vi "Load and Execute Tests Process__core.vi"(0 "TestTag Argument":string, 1 "Operation":enum16{"Load", "Run Test", "Run All Tests"}(ring), 5 "TestStatusEvents":T1, 7 "AbortEvent":refnum<user-event>, 9 "TextStream":refnum<queue>, 11 "Test Hierarchy Tree ref":refnum<vi>, 12 "API_TextTestRunner":refnum<class>, 13 "Test Project":path, 14 "error in":errorcluster) -> (4 "Tree Methods":i32, 15 "error out":errorcluster)   [LabVIEW 2013, in "GraphicalTestRunner.lvlib"]
uses:
  GraphicalTestRunner.lvlib
  Classes/TestResult/resultStatusChanged--Cluster.ctl
  Classes/TestResult/resultStatus--enum.ctl
  Classes/TestSuite/suiteStatusChanged--Cluster.ctl
  Classes/TestSuite/suiteStatus--enum.ctl
  Classes/TestSuite/TestSuite.lvclass
  Classes/TextTestRunner/TextTestRunner.lvclass
  Classes/TestLoader/TestLoader.lvclass
  Classes/TestRunner/PublicEvents--Cluster.ctl
  Classes/TestResult/testStarted--Cluster.ctl
  <userlib>/_OpenG.lib/file/file.llb/Strip Path - Arrays__ogtk.vi
  <userlib>/_OpenG.lib/array/array.llb/Filter 1D Array (String)__ogtk.vi
  <userlib>/_OpenG.lib/array/array.llb/Delete Elements from 1D Array (Path)__ogtk.vi
  <userlib>/_OpenG.lib/array/array.llb/Conditional Auto-Indexing Tunnel (Path)__ogtk.vi
  Libraries/VITesterUtilities.lvlib
  Classes/TestResult/TestResult.lvclass
  Classes/TestRunner/TestRunner.lvclass
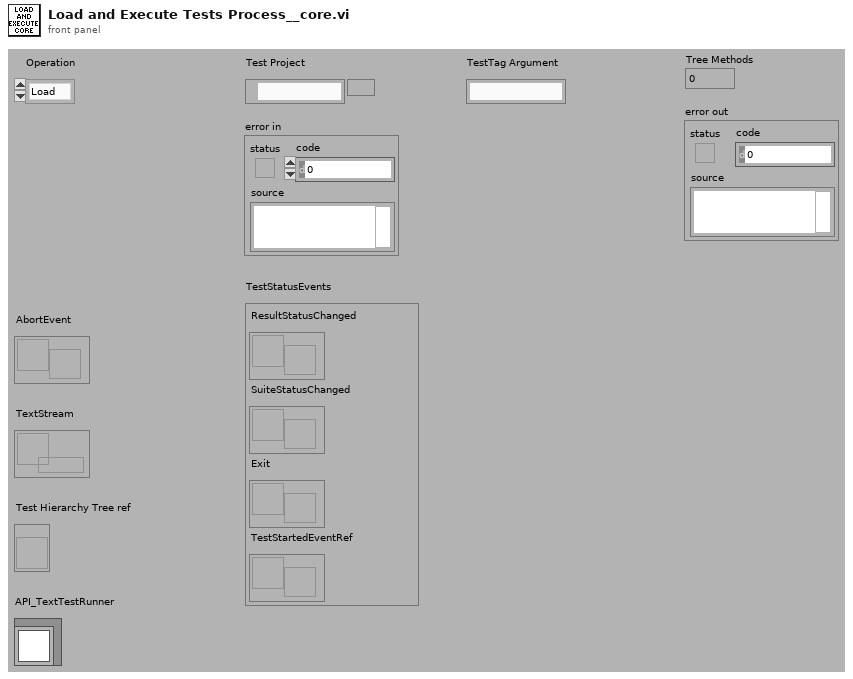
[diagram p1: front panel]
types:
  T1 = cluster{"ResultStatusChanged":refnum<user-event>, "SuiteStatusChanged":refnum<user-event>, "Exit":refnum<user-event>, "TestStartedEventRef":refnum<user-event>}
  T2 = cluster{"Current VI's Refnum":refnum<vi>, "menubar":refnum<k9>, "TextStream":refnum<queue>, "TestMethod":string, "Open Path":path, "Test Project":path, "TestProjectClasses":path[], "TestApplicationContext":refnum<vi>, "Test Class":path, "ResultChangedRef":refnum<user-event>, "SuiteChangedRef":refnum<user-event>, "TestTag":string, "AbortEventRef":refnum<user-event>, "ExitEventReference":refnum<user-event>, "AllTests.TestSuite":refnum<class "TestSuite.lvclass">, "error":errorcluster, "TextTestRunner":refnum<class "TextTestRunner.lvclass">, "TestStartedEventRef":refnum<user-event>}
  T3 = enum32{"Invalid", "Standard", "Closed", "Hidden", "Minimized", "Maximized"}
  T4 = typedef "TestRunner.lvclass/PublicEvents--Cluster.ctl" = cluster{"abortEventRef":refnum<user-event>, "resultStatusChangedEventRef":refnum<user-event>, "testStartedEventRef":refnum<user-event>}
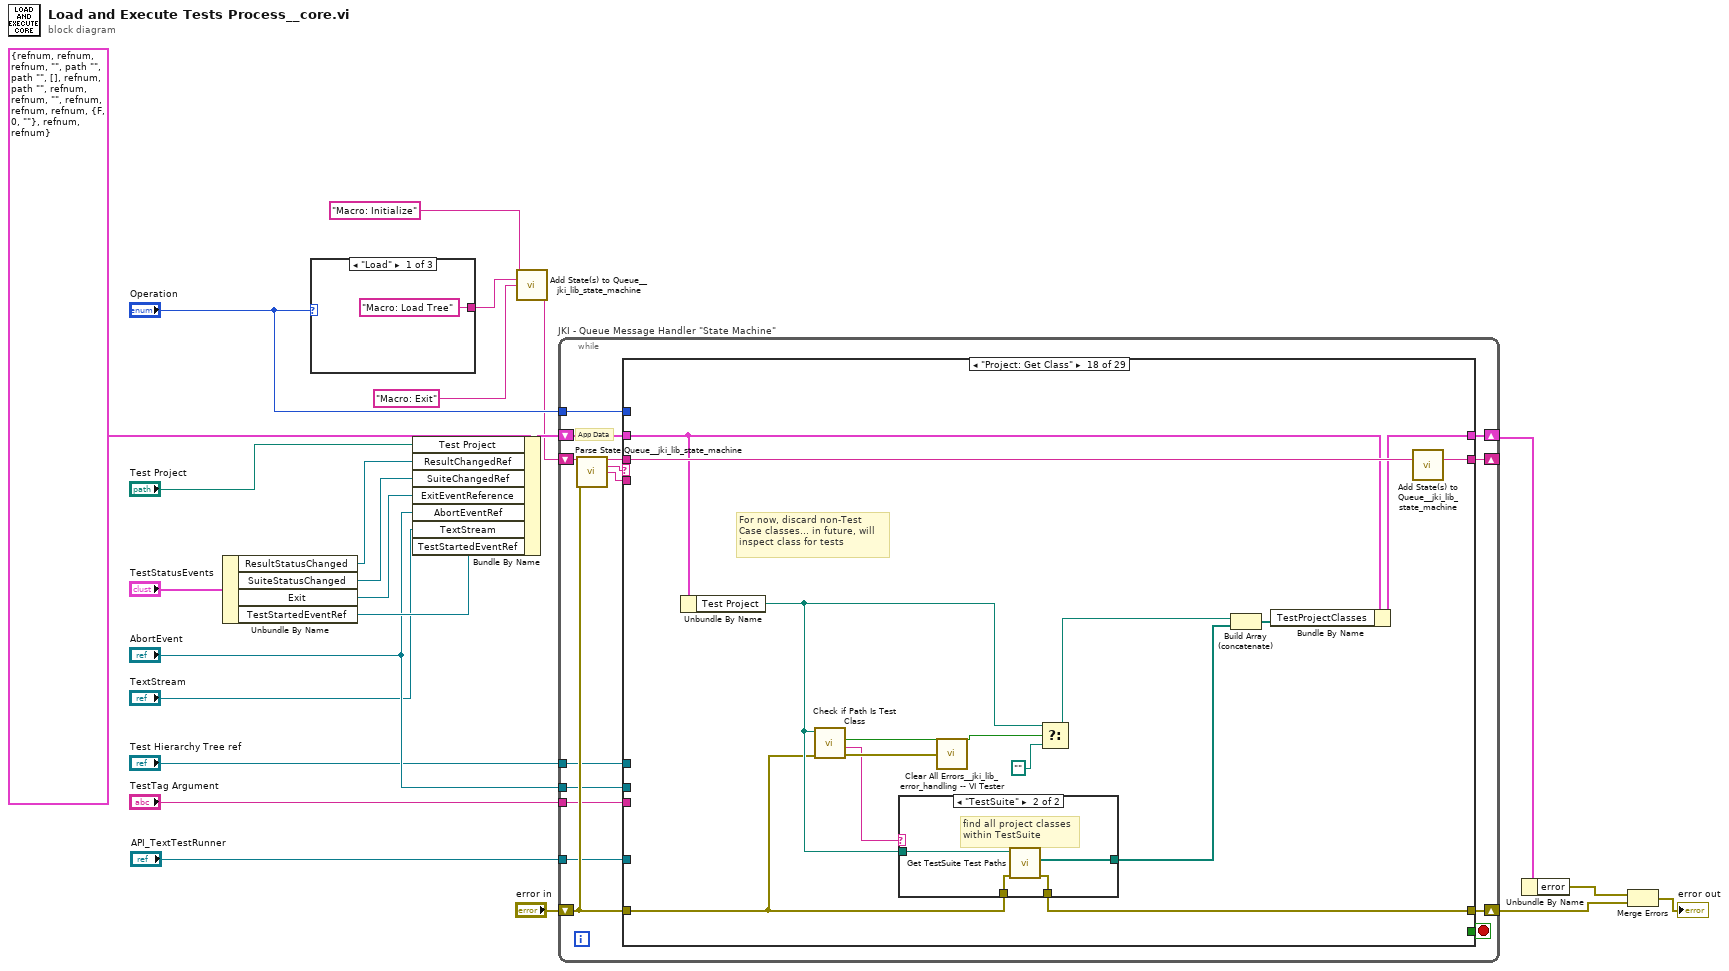
[diagram p0: block diagram]
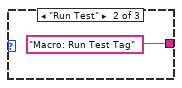
[diagram p2: hidden frame]
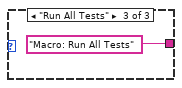
[diagram p3: hidden frame]
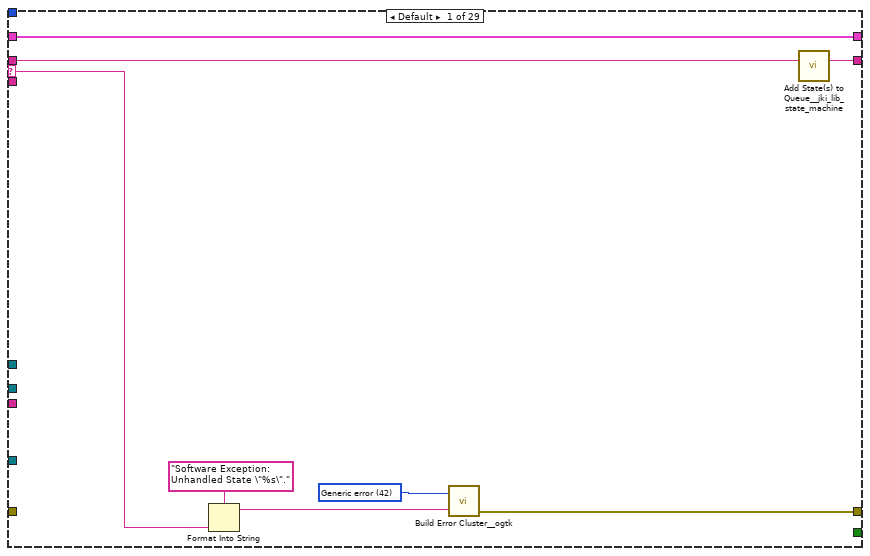
[diagram p4: hidden frame]
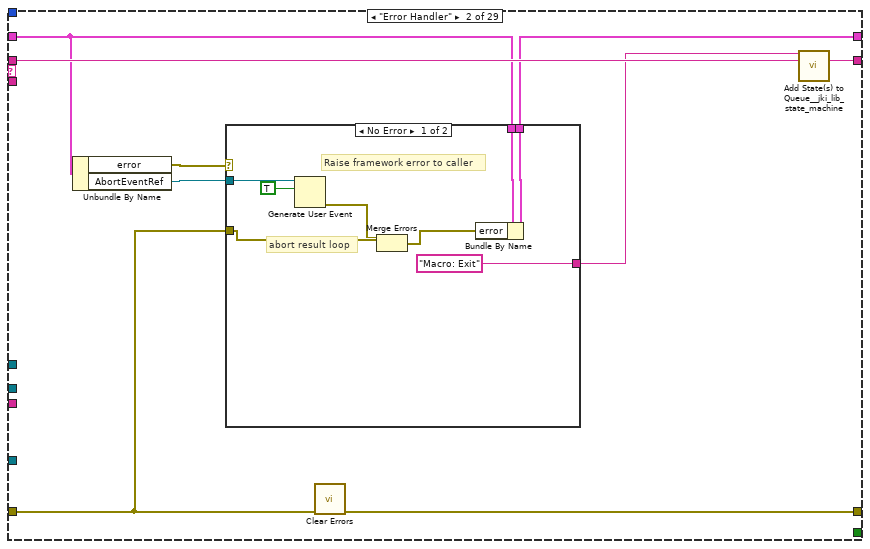
[diagram p5: hidden frame]
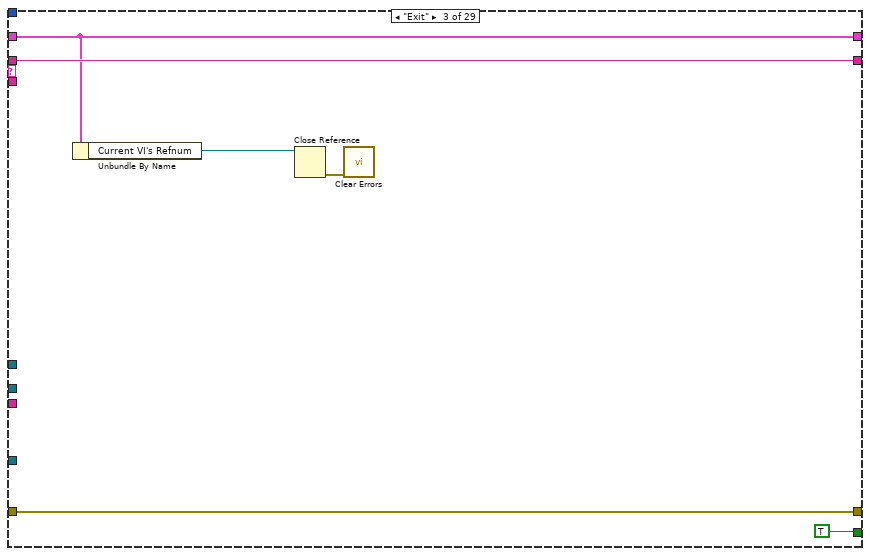
[diagram p7: hidden frame]
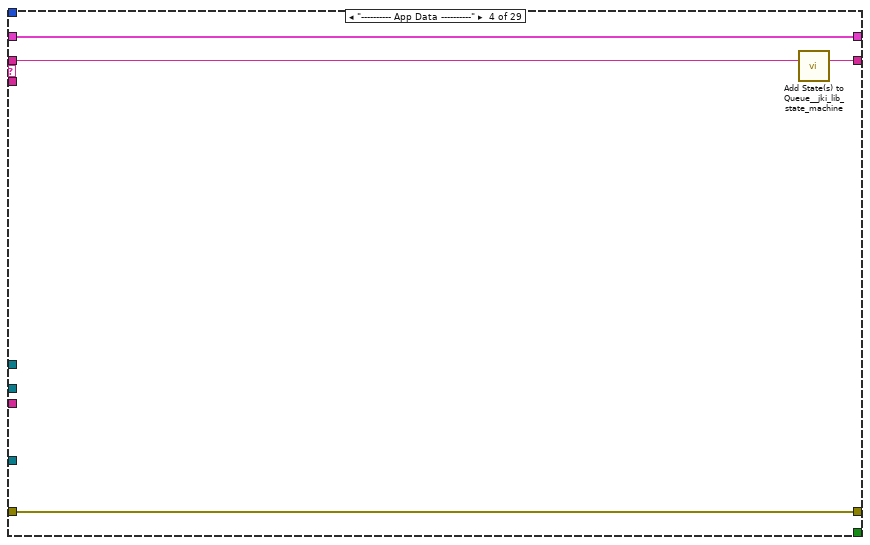
[diagram p8: hidden frame]
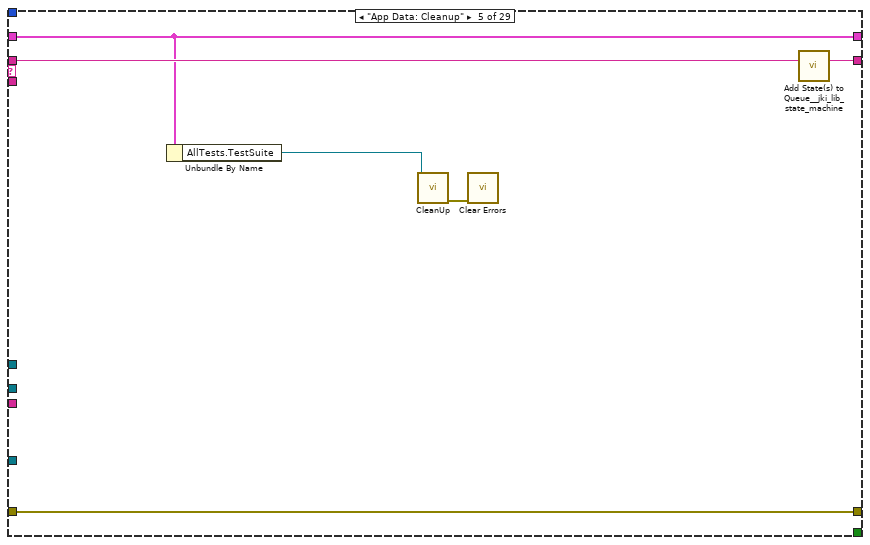
[diagram p9: hidden frame]
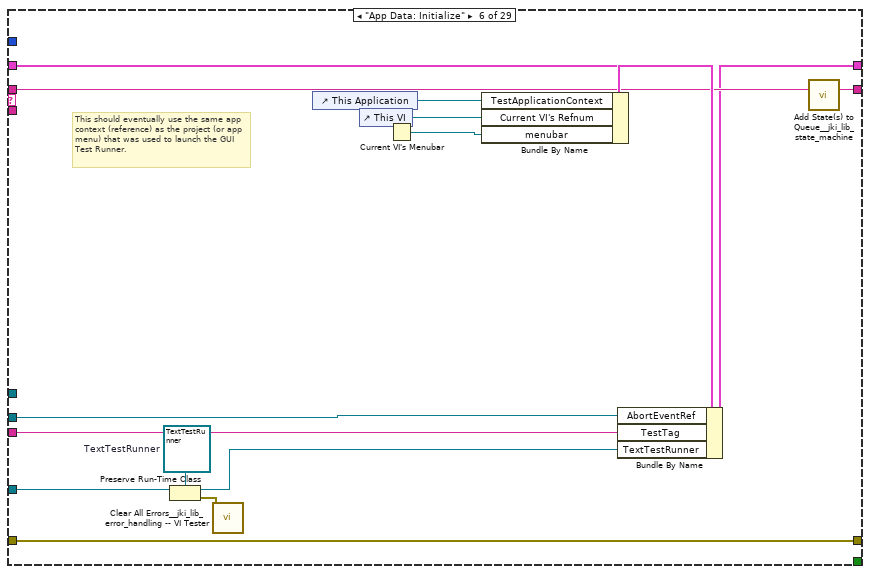
[diagram p10: hidden frame]
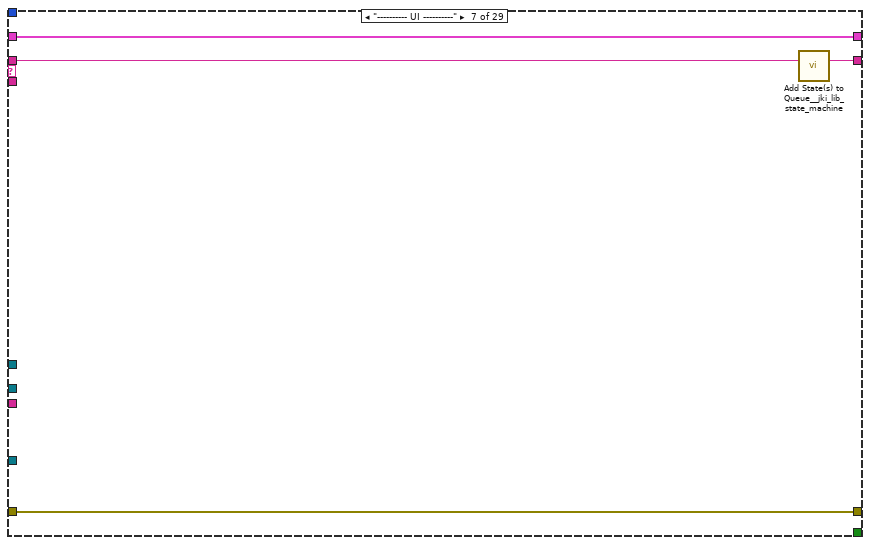
[diagram p11: hidden frame]
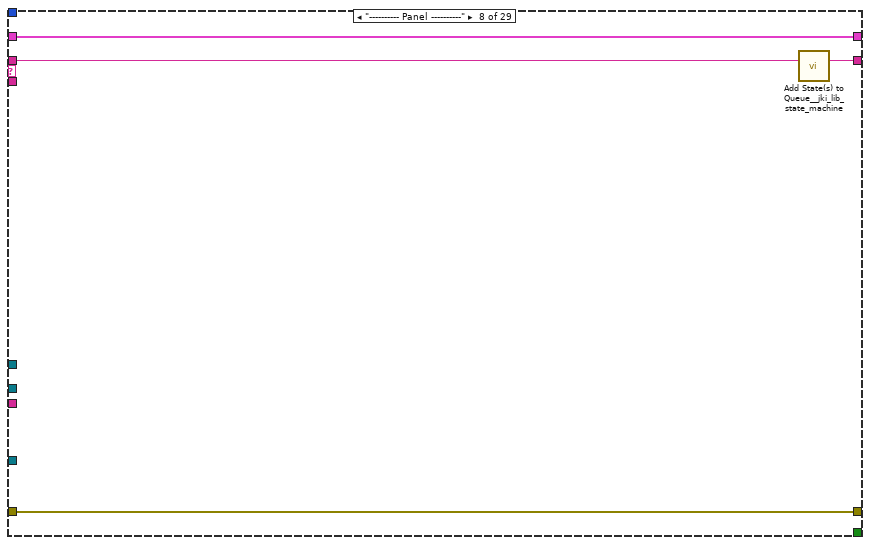
[diagram p12: hidden frame]
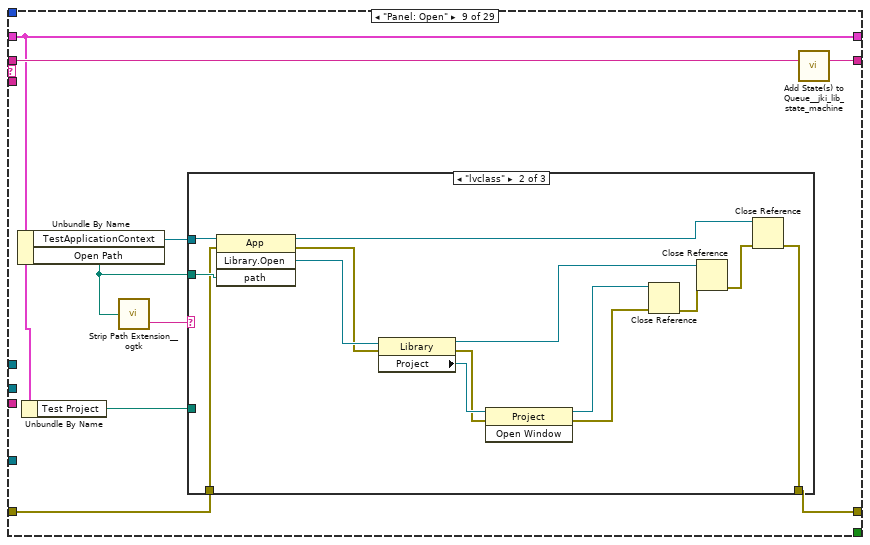
[diagram p13: hidden frame]
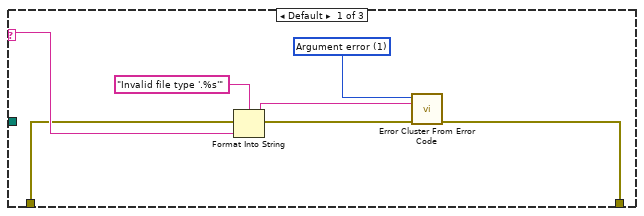
[diagram p14: hidden frame]
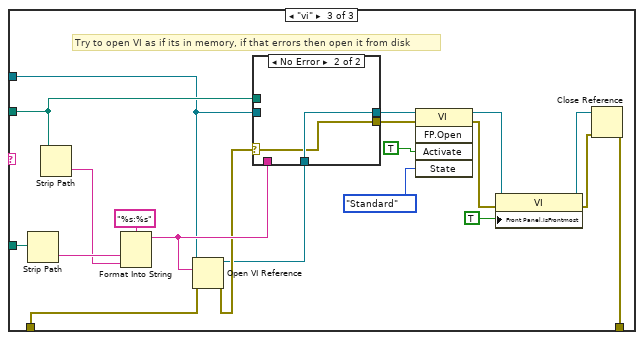
[diagram p15: hidden frame]
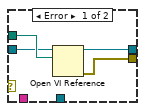
[diagram p16: hidden frame]
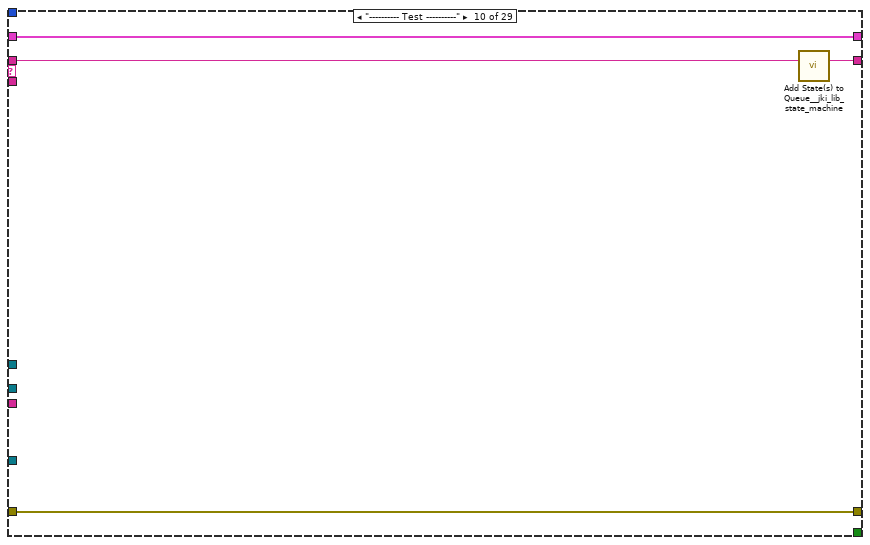
[diagram p17: hidden frame]
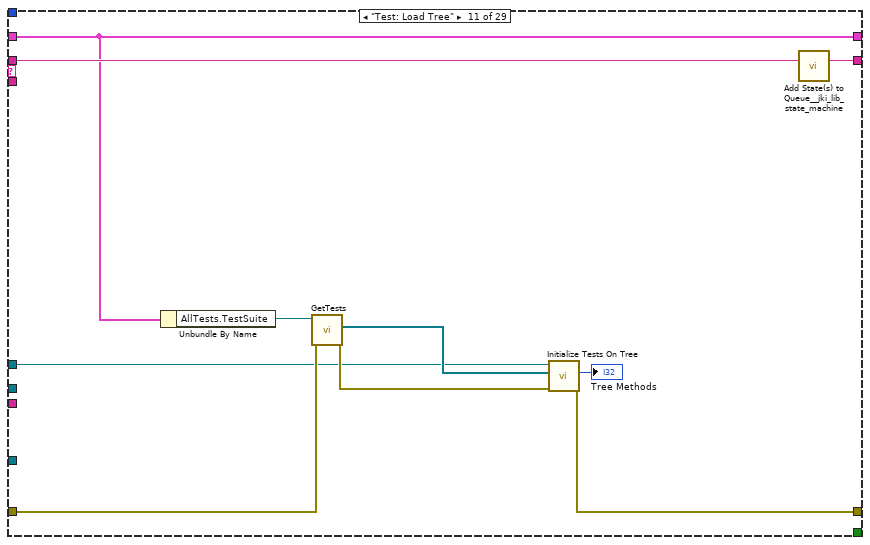
[diagram p18: hidden frame]
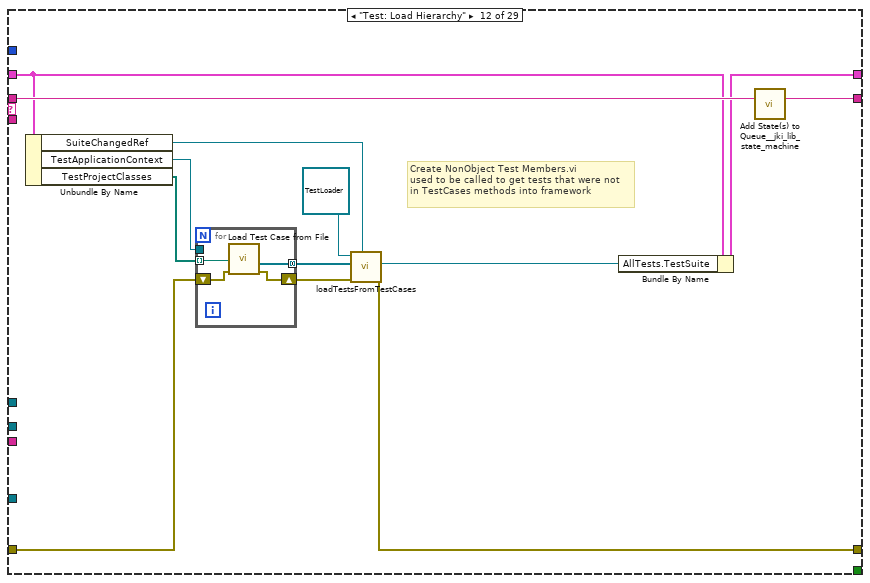
[diagram p19: hidden frame]
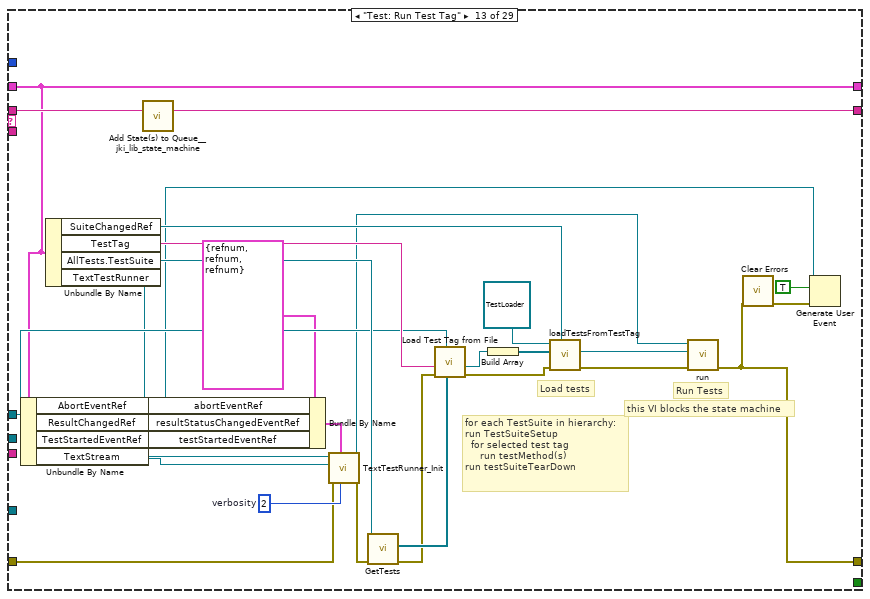
[diagram p20: hidden frame]
diagram:
  n1 = Unbundle By Name("TestStatusEvents") -> ("ResultStatusChanged"=w3:refnum<user-event>, "SuiteStatusChanged"=w4:refnum<user-event>, "Exit"=w5:refnum<user-event>, "TestStartedEventRef"=w23:refnum<user-event>)
  n2 = case shown="\"Load\"" "Operation" {
    tunnel: ["Macro: Load Tree" ("State(s) in Front") "Macro: Run Test Tag" "Macro: Run All Tests"] -> w8
    frame "Load" {
    }
    frame "Run Test" {
    }
    frame "Run All Tests" {
    }
  }
  n3 = Bundle By Name(cluster=T2 {"Current VI's Refnum"=refnum, "menubar"=refnum, "TextStream"=refnum, "TestMethod"="", "Open Path"=path "", "Test Project"=path "", "TestProjectClasses"=[], "TestApplicationContext"=refnum, "Test Class"=path "", "ResultChangedRef"=refnum, "SuiteChangedRef"=refnum, "TestTag"="", "AbortEventRef"=refnum, "ExitEventReference"=refnum, "AllTests.TestSuite"=refnum, "error"={"status"=FALSE, "code"=0, "source"=""}, "TextTestRunner"=refnum, "TestStartedEventRef"=refnum} ("SMUI Template App Data"), "Test Project"="Test Project", "ResultChangedRef"=w3, "SuiteChangedRef"=w4, "ExitEventReference"=w5, "AbortEventRef"="AbortEvent", "TextStream"="TextStream", "TestStartedEventRef"=w23) -> (w22:T2)
  n4 = call <vilib>:"Add State(s) to Queue__jki_lib_state_machine.vi"("State(s) in Front (\"\")"="Macro: Initialize", "State(s) in (\"\")"=w8, "State(s) at Back (\"\")"="Macro: Exit") -> ("States Out"=w9:string)  [unwired: 12 in]
  n5 = while "JKI - Queue Message Handler \"State Machine\"" {
    shift-right: [w41] -> w14
    shift-left: "error in" -> [w35]
    shift-right: [w39] -> _
    shift-left: w9 -> [w36]
    shift-right: [w37] -> w12
    shift-left: w22 -> [w38]
    tunnel: "Test Hierarchy Tree ref" -> [w31]
    tunnel: "Operation" -> [w30]
    tunnel: "TestTag Argument" -> [w29]
    tunnel: "AbortEvent" -> [w28]
    tunnel: "API_TextTestRunner" -> [w27]
    stop <- w40 stop-if-true
    # "App Data"
    n6 = call <vilib>:"Parse State Queue__jki_lib_state_machine.vi"("State Queue"=w36, "Error In (no error)"=w35) -> ("Remaining States"=w34:string, "Current State"=w32:string, "Arguments"=w33:string)  [unwired: 11 in]
    n7 = case shown="\"Project: Get Class\"" w32 {
      selector: w32 -> [w48 _ _ _ _ _ _ _ _ _ _ _ _ _ _ _ _ _ _ _ _ _ _ _ _ _ _ _ _]
      tunnel: w34 -> [w46 w58 w71 w75 w83 w97 w100 w104 w115 w163 w175 w188 w221 w239 w241 w244 w256 w290 w297 w304 w313 w326 w331 w337 w341 w345 w356 w366 w368]
      tunnel: [w42 w51 w73 w77 w79 w95 w102 w106 w108 w165 w168 w176 w198 w227 w243 w246 w252 w278 w299 w301 w306 w328 w333 w338 w343 w347 w350 w361 w370] -> w41
      tunnel: w35 -> [_ w52 w73 w77 w79 w95 w102 w106 w109 w165 w169 w185 w204 w233 w243 w246 w254 w279 w299 w301 w307 w328 w333 w338 w343 w347 _ w362 w370]
      tunnel: [_ _ TRUE _ _ _ _ _ _ _ _ _ _ _ _ _ _ _ _ _ _ _ _ _ _ _ _ _ _] -> w40
      tunnel: [w47 w57 w71 w74 w82 w96 w99 w103 w114 w162 w174 w187 w220 w238 w240 w244 w255 w289 w296 w303 w312 w325 w330 w336 w340 w344 w355 w365 w367] -> w39
      tunnel: w38 -> [w45 w55 w70 w76 w81 w86 w101 w105 w111 w164 w166 w186 w201 w230 w242 w245 w251 w287 w298 w302 w308 w327 w332 w335 w342 w346 w349 w358 w369]
      tunnel: [w45 w54 w70 w76 w81 w94 w101 w105 w111 w164 w166 w184 w201 w230 w242 w245 w253 w288 w298 w302 w308 w327 w332 w335 w342 w346 w349 w360 w369] -> w37
      tunnel: w33 -> [_ _ _ _ _ _ _ _ _ _ _ _ _ _ _ _ _ _ _ _ _ _ _ _ _ _ _ _ _]
      tunnel: w31 -> [_ _ _ _ _ _ _ _ _ _ w167 _ w212 _ _ _ _ _ _ _ _ _ _ _ _ _ _ _ _]
      tunnel: w30 -> [_ _ _ _ _ _ _ _ _ _ _ _ _ _ _ _ _ _ _ _ _ _ _ _ _ _ _ _ _]
      tunnel: w29 -> [_ _ _ _ _ w93 _ _ _ _ _ _ _ _ _ _ _ _ _ _ _ _ _ _ _ _ _ _ _]
      tunnel: w28 -> [_ _ _ _ _ w92 _ _ _ _ _ _ _ _ _ _ _ _ _ _ _ _ _ _ _ _ _ _ _]
      tunnel: w27 -> [_ _ _ _ _ w91 _ _ _ _ _ _ _ _ _ _ _ _ _ _ _ _ _ _ _ _ _ _ _]
      frame Default {
        w44 = 42 items=["No error", "Argument error", "Memory is full", "Out of zone", "End of file", "File already open", "Generic file I/O error", "File not found", "File permission error", "Disk is full", "Duplicate path", "Too many files open", "System feature not enabled", "Resource file not found", "Cannot add resource", "Resource not found", "Image not found", "Image memory error", "Pen does not exist", "Config type invalid", "Config token not found", "Config parse error", "Config memory error", "Bad external code format", "Bad external code offset", "External code not present", "Null window", "Destroy window error", "Null menu", "Print aborted", "Bad print record", "Print driver error", "Windows error during printing", "Memory error during printing", "Print dialog error", "Generic print error", "Invalid device refnum", "Device not found", "Device parameter error", "Device unit error", "Cannot open device", "Device call aborted", "Generic error", "Cancelled by user", "Object ID too low", "Object ID too high", "Object not in heap", "Unknown heap", "Unknown object (invalid DefProc)", "Unknown object (DefProc not in table)", "Message out of range", "Invalid (null) method", "Unknown message", "Manager call not supported", "Bad address", "Network operation in progress", "Network operation timed out", "Connection is busy", "Network attribute not supported", "Network error", "Address in use", "System out of memory", "Connection aborted", "Connection refused", "Not connected", "Already connected", "Connection closed", "Initialization error (interapplication manager)", "Bad occurrence", "Wait on unbound occurrence handler", "Occurrence queue overflow", "Datalog type conflict", "Unused", "Unrecognized type (interapplication manager)", "Memory corrupt", "Failed to make temporary DLL", "Old CIN version", "Drag socket not found", "Failed to load drop-object", "Failed to register OLE object", "Failed to release OLE object", "Format specifier type mismatch", "Unknown format specifier", "Too few format specifiers", "Too many format specifiers", "Scan failed", "Newer CIN version", "Error converting to variant", "Runtime menu error", "Password tampered", "Variant attribute not found", "Incompatible variant data type", "Event data is not available", "Event Store is not present", "Occurrence is not found", "Event Queue is not created", "Event info is not available", "Refnum passed is NULL", "Error retrieving Class GUID", "Error retrieving CoClass GUID", "Error retrieving TypeLib GUID.", "Bad built application magic bytes.", "Specific driver is different from the specific driver associated with the Logical Name.", "There is no session opened to the class driver.", "Max Error", "MAX - Error with config objects", "MAX - Error loading configuration", "MAX - Group not supported"]
        n8 = Format Into String(format string="Software Exception: Unhandled State \"%s\"." ("message"), w48) -> (resulting string=w43:string)  [unwired: 2 in, 1 out]
        n9 = call <userlib>:"Build Error Cluster__ogtk.vi"("String to Prepend to source (\"\")"=w43, "code"=w44) -> ("error out"=w42:errorcluster)
        n10 = call <vilib>:"Add State(s) to Queue__jki_lib_state_machine.vi"("State(s) in (\"\")"=w46) -> ("States Out"=w47:string)  [unwired: 14 in]
      }
      frame "Error Handler" {
        n11 = Unbundle By Name(w55) -> ("error"=w53:errorcluster, "AbortEventRef"=w50:refnum<user-event>)
        n12 = case shown="No Error" w53 {
          tunnel: ["Macro: Exit" ("State(s) in Front (\"\")") _] -> w56
          tunnel: w55 -> [w65 w67]
          tunnel: [w64 w67] -> w54
          tunnel: w52 -> [w61 _]
          tunnel: w50 -> [w63 _]
          frame No Error {
            # "abort result loop"
            # "Raise framework error to caller"
            n13 = Generate User Event(user event=w63, event data cluster=TRUE ("event data")) -> (error out=w60:errorcluster)  [unwired: 2 in, 1 out]
            n14 = Merge Errors(w61, w60) -> (w59:errorcluster)
            n15 = Bundle By Name(cluster=w65, "error"=w59) -> (w64:T2)
          }
          frame Error {
          }
        }
        n16 = call <vilib>:"Clear Errors.vi"("error in (no error)"=w52) -> ("error out"=w51:errorcluster)  [unwired: 6 in]
        n17 = call <vilib>:"Add State(s) to Queue__jki_lib_state_machine.vi"("State(s) in Front (\"\")"=w56, "State(s) in (\"\")"=w58) -> ("States Out"=w57:string)  [unwired: 13 in]
      }
      frame "Exit" {
        n18 = Unbundle By Name(w70) -> ("Current VI's Refnum"=w69:refnum<vi>)
        n19 = Close Reference(reference=w69) -> (error out=w68:errorcluster)  [unwired: 1 in]
        n20 = call <vilib>:"Clear Errors.vi"("error in (no error)"=w68) -> ()  [unwired: 6 in, 1 out]
      }
      frame "---------- App Data ----------" {
        n21 = call <vilib>:"Add State(s) to Queue__jki_lib_state_machine.vi"("State(s) in (\"\")"=w75) -> ("States Out"=w74:string)  [unwired: 14 in]
      }
      frame "App Data: Cleanup" {
        n22 = Unbundle By Name(w81) -> ("AllTests.TestSuite"=w78:refnum<class "TestSuite.lvclass">)
        n23 = call-dynamic "CleanUp.vi"("TestSuite in"=w78) -> ("error out"=w80:errorcluster)  [unwired: 9 in, 1 out]
        n24 = call <vilib>:"Clear Errors.vi"("error in (no error)"=w80) -> ()  [unwired: 6 in, 1 out]
        n25 = call <vilib>:"Add State(s) to Queue__jki_lib_state_machine.vi"("State(s) in (\"\")"=w83) -> ("States Out"=w82:string)  [unwired: 14 in]
      }
      frame "App Data: Initialize" {
        w90 = refnum<class "TextTestRunner.lvclass"> refnum  # TextTestRunner
        # "This should eventually use the same app context (reference) as the project (or app menu) that was used to launch the GUI Test Runner."
        n26 = Preserve Run-Time Class(object in=w91, 2:w90) -> (object out=w89:refnum<class "TextTestRunner.lvclass">, error out=w88:errorcluster)  [unwired: 1 in]
        n27 = call "Clear All Errors__jki_lib_error_handling -- VI Tester.vi"("error in"=w88) -> ()  [unwired: 4 in, 1 out]
        n28 = control-ref of="This Application"() -> (w85:refnum<vi>)
        n29 = control-ref of="This VI"() -> (w84:refnum<vi>)
        n30 = Current VI's Menubar() -> (w87:refnum<k9>)
        n31 = Bundle By Name(cluster=w86, "TestApplicationContext"=w85, "Current VI's Refnum"=w84, "menubar"=w87) -> (w98:T2)
        n32 = Bundle By Name(cluster=w98, "AbortEventRef"=w92, "TestTag"=w93, "TextTestRunner"=w89) -> (w94:T2)
        n33 = call <vilib>:"Add State(s) to Queue__jki_lib_state_machine.vi"("State(s) in (\"\")"=w97) -> ("States Out"=w96:string)  [unwired: 14 in]
      }
      frame "---------- UI ----------" {
        n34 = call <vilib>:"Add State(s) to Queue__jki_lib_state_machine.vi"("State(s) in (\"\")"=w100) -> ("States Out"=w99:string)  [unwired: 14 in]
      }
      frame "---------- Panel ----------" {
        n35 = call <vilib>:"Add State(s) to Queue__jki_lib_state_machine.vi"("State(s) in (\"\")"=w104) -> ("States Out"=w103:string)  [unwired: 14 in]
      }
      frame "Panel: Open" {
        n36 = Unbundle By Name(w111) -> ("TestApplicationContext"=w107:refnum<vi>, "Open Path"=w112:path)
        n37 = Unbundle By Name(w111) -> ("Test Project"=w110:path)
        n38 = call-poly <userlib>:"Strip Path Extension__ogtk.vi"("path"=w112) -> ("extension"=w113:string)  [unwired: 1 out]
        n39 = case shown="\"lvclass\"" w113 {
          selector: w113 -> [w119 _ _]
          tunnel: w112 -> [_ w135 w146]
          tunnel: w110 -> [_ _ w149]
          tunnel: w109 -> [w116 w134 w139]
          tunnel: [w117 w123 w148] -> w108
          tunnel: w107 -> [_ w122 w138]
          frame Default {
            w121 = 1 items=["No error", "Argument error", "Memory is full", "Out of zone", "End of file", "File already open", "Generic file I/O error", "File not found", "File permission error", "Disk is full", "Duplicate path", "Too many files open", "System feature not enabled", "Resource file not found", "Cannot add resource", "Resource not found", "Image not found", "Image memory error", "Pen does not exist", "Config type invalid", "Config token not found", "Config parse error", "Config memory error", "Bad external code format", "Bad external code offset", "External code not present", "Null window", "Destroy window error", "Null menu", "Print aborted", "Bad print record", "Print driver error", "Windows error during printing", "Memory error during printing", "Print dialog error", "Generic print error", "Invalid device refnum", "Device not found", "Device parameter error", "Device unit error", "Cannot open device", "Device call aborted", "Generic error", "Cancelled by user", "Object ID too low", "Object ID too high", "Object not in heap", "Unknown heap", "Unknown object (invalid DefProc)", "Unknown object (DefProc not in table)", "Message out of range", "Invalid (null) method", "Unknown message", "Manager call not supported", "Bad address", "Network operation in progress", "Network operation timed out", "Connection is busy", "Network attribute not supported", "Network error", "Address in use", "System out of memory", "Connection aborted", "Connection refused", "Not connected", "Already connected", "Connection closed", "Initialization error (interapplication manager)", "Bad occurrence", "Wait on unbound occurrence handler", "Occurrence queue overflow", "Datalog type conflict", "Unused", "Unrecognized type (interapplication manager)", "Memory corrupt", "Failed to make temporary DLL", "Old CIN version", "Drag socket not found", "Failed to load drop-object", "Failed to register OLE object", "Failed to release OLE object", "Format specifier type mismatch", "Unknown format specifier", "Too few format specifiers", "Too many format specifiers", "Scan failed", "Newer CIN version", "Error converting to variant", "Runtime menu error", "Password tampered", "Variant attribute not found", "Incompatible variant data type", "Event data is not available", "Event Store is not present", "Occurrence is not found", "Event Queue is not created", "Event info is not available", "Refnum passed is NULL", "Error retrieving Class GUID", "Error retrieving CoClass GUID", "Error retrieving TypeLib GUID.", "Bad built application magic bytes.", "Specific driver is different from the specific driver associated with the Logical Name.", "There is no session opened to the class driver.", "Max Error", "MAX - Error with config objects", "MAX - Error loading configuration", "MAX - Group not supported"]
            n40 = Format Into String(format string="Invalid file type '.%s'", w119) -> (resulting string=w118:string)  [unwired: 2 in, 1 out]
            n41 = call <vilib>:"Error Cluster From Error Code.vi"("error in (no error)"=w116, "error message (\"\")"=w118, "error code (0)"=w121) -> ("error out"=w117:errorcluster)  [unwired: 6 in]
          }
          frame "lvclass" {
            n42 = invoke class="App" method="Library.Open"(reference=w122, error in=w134, "path"=w135) -> (reference out=w127:refnum<vi>, error out=w130:errorcluster, "Open Library"=w133:refnum<vi>)  [unwired: 1 in, 1 out]
            n43 = property class="Library"(reference=w133, error in=w130) -> (reference out=w128:refnum<vi>, error out=w131:errorcluster, "Project"=w132:refnum<vi>)
            n44 = invoke class="Project" method="Open Window"(reference=w132, error in=w131) -> (reference out=w129:refnum<vi>, error out=w124:errorcluster)  [unwired: 1 in, 1 out]
            n45 = Close Reference(reference=w129, error in (no error)=w124) -> (error out=w126:errorcluster)
            n46 = Close Reference(reference=w128, error in (no error)=w126) -> (error out=w125:errorcluster)
            n47 = Close Reference(reference=w127, error in (no error)=w125) -> (error out=w123:errorcluster)
          }
          frame "vi" {
            # "Try to open VI as if its in memory, if that errors then open it from disk"
            n48 = Strip Path(path=w149) -> (name=w155:string)  [unwired: 1 out]
            n49 = Strip Path(path=w146) -> (name=w154:string)  [unwired: 1 out]
            n50 = Format Into String(format string="%s:%s", w155, w154) -> (resulting string=w140:string)  [unwired: 2 in, 1 out]
            n51 = Open VI Reference(application reference (local)=w138, vi path=w140, error in (no error)=w139) -> (vi reference=w136:refnum<vi>, error out=w137:errorcluster)  [unwired: 3 in]
            n52 = case shown="No Error" w137 {
              selector: w137 -> [_ w160]
              tunnel: [w159 w160] -> w151
              tunnel: [w158 w161] -> w150
              tunnel: w140 -> [_ _]
              tunnel: w146 -> [w157 _]
              tunnel: w138 -> [w156 _]
              tunnel: w136 -> [_ w161]
              frame Error {
                n53 = Open VI Reference(application reference (local)=w156, vi path=w157) -> (vi reference=w158:refnum<vi>, error out=w159:errorcluster)  [unwired: 4 in]
              }
              frame No Error {
              }
            }
            n54 = invoke class="VI" method="FP.Open"(reference=w150, error in=w151, "Activate"=TRUE ("Activate?"), "State"=T3."Standard") -> (reference out=w142:refnum<vi>, error out=w144:errorcluster)  [unwired: 1 in, 3 out]
            n55 = property class="VI"(reference=w142, error in=w144, "Front Panel.IsFrontmost"=TRUE ("Front Panel Window:Is Frontmost")) -> (reference out=w141:refnum<vi>, error out=w143:errorcluster)
            n56 = Close Reference(reference=w141, error in (no error)=w143) -> (error out=w148:errorcluster)
          }
        }
        n57 = call <vilib>:"Add State(s) to Queue__jki_lib_state_machine.vi"("State(s) in (\"\")"=w115) -> ("States Out"=w114:string)  [unwired: 14 in]
      }
      frame "---------- Test ----------" {
        n58 = call <vilib>:"Add State(s) to Queue__jki_lib_state_machine.vi"("State(s) in (\"\")"=w163) -> ("States Out"=w162:string)  [unwired: 14 in]
      }
      frame "Test: Load Tree" {
        n59 = Unbundle By Name(w166) -> ("AllTests.TestSuite"=w170:refnum<class "TestSuite.lvclass">)
        n60 = call-dynamic "GetTests.vi"("error in (no error)"=w169, "TestSuite in"=w170) -> ("error out"=w173:errorcluster, "tests"=w172:refnum<class>[])  [unwired: 7 in, 1 out]
        n61 = call "Initialize Tests On Tree.vi"("error in"=w173, "tests"=w172, "Tree reference"=w167) -> ("error out"=w168:errorcluster, "Tree Methods"=→"Tree Methods":i32)  [unwired: 7 in]
        n62 = call <vilib>:"Add State(s) to Queue__jki_lib_state_machine.vi"("State(s) in (\"\")"=w175) -> ("States Out"=w174:string)  [unwired: 14 in]
      }
      frame "Test: Load Hierarchy" {
        # "Create NonObject Test Members.vi\nused to be called to get tests that were not\nin TestCases methods into framework"
        n63 = Unbundle By Name(w186) -> ("SuiteChangedRef"=w178:refnum<user-event>, "TestApplicationContext"=w182:refnum<vi>, "TestProjectClasses"=w183:path[])
        n64 = for {
          tunnel: [w190] -> w181 mode=concatenating
          tunnel: w182 -> [_]
          tunnel: w183 -> [w189] mode=indexing
          shift-right: [w191] -> w180
          shift-left: w185 -> [w192]
          n65 = call "Load Test Case from File.vi"("error in"=w192, "Test Class Path"=w189) -> ("error out"=w191:errorcluster, "Test Case"=w190:refnum<class>[])  [unwired: 8 in]
        }
        n66 = call-dynamic "loadTestsFromTestCases.vi"("testSuiteStatusChangedRef"=w178, "error in (no error)"=w180, "Tests"=w181, "TestLoader in"=refnum<class "TestLoader.lvclass"> refnum ("reference in")) -> ("error out"=w176:errorcluster, "TestSuite"=w177:refnum<class "TestSuite.lvclass">)  [unwired: 5 in, 1 out]
        n67 = Bundle By Name(cluster=w186, "AllTests.TestSuite"=w177) -> (w184:T2)
        n68 = call <vilib>:"Add State(s) to Queue__jki_lib_state_machine.vi"("State(s) in (\"\")"=w188) -> ("States Out"=w187:string)  [unwired: 14 in]
      }
      frame "Test: Run Test Tag" {
        w208 = u32 2  # verbosity
        # "Load tests"
        # "for each TestSuite in hierarchy:\nrun TestSuiteSetup\n  for selected test tag\n     run testMethod(s)\nrun testSuiteTearDown"
        # "this VI blocks the state machine"
        # "Run Tests"
        n69 = Unbundle By Name(w201) -> ("AbortEventRef"=w200:refnum<user-event>, "ResultChangedRef"=w207:refnum<user-event>, "TestStartedEventRef"=w193:refnum<user-event>, "TextStream"=w205:refnum<queue>)
        n70 = Unbundle By Name(w201) -> ("SuiteChangedRef"=w218:refnum<user-event>, "TestTag"=w217:string, "AllTests.TestSuite"=w216:refnum<class "TestSuite.lvclass">, "TextTestRunner"=w194:refnum<class "TextTestRunner.lvclass">)
        n71 = call <vilib>:"Add State(s) to Queue__jki_lib_state_machine.vi"("State(s) in (\"\")"=w221) -> ("States Out"=w220:string)  [unwired: 14 in]
        n72 = Bundle By Name(cluster=T4 {"abortEventRef"=refnum, "resultStatusChangedEventRef"=refnum, "testStartedEventRef"=refnum} ("publicEvents"), "abortEventRef"=w200, "resultStatusChangedEventRef"=w207, "testStartedEventRef"=w193) -> (w206:T4)
        n73 = call "TextTestRunner_Init.vi"("verbosity (1)"=w208, "publicEvents"=w206, "error in (no error)"=w204, "stream"=w205, "TextTestRunner in"=w194) -> ("error out"=w203:errorcluster, "TextTestRunner out"=w202:refnum<class "TextTestRunner.lvclass">)  [unwired: 5 in]
        n74 = call-dynamic "GetTests.vi"("error in (no error)"=w203, "TestSuite in"=w216) -> ("error out"=w214:errorcluster, "tests"=w215:refnum<class>[])  [unwired: 7 in, 1 out]
        n75 = call "Load Test Tag from File.vi"("AllTests"=w215, "Tree reference"=w212, "error in"=w214, "TestTag"=w217) -> ("error out"=w210:errorcluster, "Test Tag Test"=w209:refnum<class>)  [unwired: 6 in]
        n76 = Build Array(w209) -> (w195:refnum<class>[])
        n77 = call-dynamic "loadTestsFromTestTag.vi"("testSuiteStatusChangedRef"=w218, "error in (no error)"=w210, "Tests"=w195, "TestLoader in"=refnum<class "TestLoader.lvclass"> refnum ("reference in")) -> ("error out"=w213:errorcluster, "TestSuite"=w219:refnum<class "TestSuite.lvclass">)  [unwired: 5 in, 1 out]
        n78 = call-dynamic "run.vi"("error in (no error)"=w213, "test"=w219, "TextTestRunner in"=w202) -> ("error out"=w198:errorcluster)  [unwired: 6 in, 2 out]
        n79 = call <vilib>:"Clear Errors.vi"("error in (no error)"=w198) -> ("error out"=w197:errorcluster)  [unwired: 6 in]
        n80 = Generate User Event(user event=w200, event data cluster=TRUE ("event data"), error in=w197) -> ()  [unwired: 1 in, 2 out]
      }
      frame "Test: Run All Tests" {
        w236 = u32 2  # verbosity
        # "Run Tests"
        n81 = Unbundle By Name(w230) -> ("AllTests.TestSuite"=w237:refnum<class "TestSuite.lvclass">)
        n82 = Unbundle By Name(w230) -> ("AbortEventRef"=w228:refnum<user-event>, "ResultChangedRef"=w235:refnum<user-event>, "TestStartedEventRef"=w222:refnum<user-event>, "TextStream"=w234:refnum<queue>, "TextTestRunner"=w223:refnum<class "TextTestRunner.lvclass">)
        n83 = Bundle By Name(cluster=T4 {"abortEventRef"=refnum, "resultStatusChangedEventRef"=refnum, "testStartedEventRef"=refnum} ("publicEvents"), "abortEventRef"=w228, "resultStatusChangedEventRef"=w235, "testStartedEventRef"=w222) -> (w224:T4)
        n84 = call "TextTestRunner_Init.vi"("verbosity (1)"=w236, "publicEvents"=w224, "error in (no error)"=w233, "stream"=w234, "TextTestRunner in"=w223) -> ("error out"=w232:errorcluster, "TextTestRunner out"=w231:refnum<class "TextTestRunner.lvclass">)  [unwired: 5 in]
        n85 = call-dynamic "run.vi"("error in (no error)"=w232, "test"=w237, "TextTestRunner in"=w231) -> ("error out"=w227:errorcluster)  [unwired: 6 in, 2 out]
        n86 = call <vilib>:"Clear Errors.vi"("error in (no error)"=w227) -> ("error out"=w226:errorcluster)  [unwired: 6 in]
        n87 = Generate User Event(user event=w228, event data cluster=TRUE ("event data"), error in=w226) -> ()  [unwired: 1 in, 2 out]
        n88 = call <vilib>:"Add State(s) to Queue__jki_lib_state_machine.vi"("State(s) in (\"\")"=w239) -> ("States Out"=w238:string)  [unwired: 14 in]
      }
      frame "---------- Project ----------" {
        n89 = call <vilib>:"Add State(s) to Queue__jki_lib_state_machine.vi"("State(s) in (\"\")"=w241) -> ("States Out"=w240:string)  [unwired: 14 in]
      }
      frame "Project: Get Tests" {
        # "no longer support tests outside of testCase objects"
      }
      frame "Project: Get Classes" {
        n90 = Unbundle By Name(w251) -> ("TestApplicationContext"=w250:refnum<vi>)
        n91 = Unbundle By Name(w251) -> ("Test Project"=w248:path)
        n92 = call-poly <userlib>:"Strip Path Extension__ogtk.vi"("path"=w248) -> ("extension"=w247:string)  [unwired: 1 out]
        n93 = case "Load Project from lvproj file" shown="\"lvproj\"" w247 {
          tunnel: w254 -> [w266 w276]
          tunnel: [w261 w275] -> w252
          tunnel: w250 -> [w262 _]
          tunnel: [w258 w273] -> w249
          tunnel: w248 -> [w267 w274]
          frame Default {
            w257 = string[] ["TestCase.lvclass", "TestSuite.lvclass"]  # Framework classes
            # "load from folder -- find all *.lvclass that are not part of the framework"
            n94 = call <userlib>:"List Directory Recursive__ogtk.vi"("error in (no error)"=w266, "pattern"="*.lvclass", "Path"=w267) -> ("error out"=w261:errorcluster, "file paths"=w263:path[])  [unwired: 5 in, 2 out]
            n95 = call-poly <userlib>:"Strip Path__ogtk.vi"("path"=w263) -> ("name"=w265:string[])  [unwired: 1 out]
            n96 = call-poly <userlib>:"Filter 1D Array__ogtk.vi"("items to filter"=w257, "array"=w265) -> ("filtered item indices"=w264:i32[])  [unwired: 4 in, 1 out]
            n97 = call-poly <userlib>:"Delete Elements from Array__ogtk.vi"("indices"=w264, "array"=w263) -> ("array w/ subset deleted"=w259:path[])  [unwired: 8 in, 1 out]
            n98 = for {
              tunnel: w262 -> [_]
              tunnel: w259 -> [w272] mode=indexing
              tunnel: w261 -> [w271]
              tunnel: [w270] -> w260 mode=indexing
              n99 = call "Check if Path Is Test Class.vi"("error in"=w271, "Test Class Path"=w272) -> ("error out"=w269:errorcluster, "IsTestObject"=w270:bool)  [unwired: 7 in, 1 out]
              n100 = call <vilib>:"Clear Errors.vi"("error in (no error)"=w269) -> ()  [unwired: 6 in, 1 out]
            }
            n101 = call-poly <userlib>:"Conditional Auto-Indexing Tunnel__ogtk.vi"("Array in"=w259, "Elements to keep"=w260) -> ("Filtered Array out"=w258:path[])  [unwired: 5 in]
          }
          frame "lvproj" {
            n102 = call "Find Project Test Objects.vi"("error in"=w276, "Project"=w274) -> ("error out"=w275:errorcluster, "TestPaths"=w273:path[])  [unwired: 8 in]
          }
        }
        n103 = Bundle By Name(cluster=w251, "TestProjectClasses"=w249) -> (w253:T2)
        n104 = call <vilib>:"Add State(s) to Queue__jki_lib_state_machine.vi"("State(s) in (\"\")"=w256) -> ("States Out"=w255:string)  [unwired: 14 in]
      }
      frame "Project: Get Class" {
        # "For now, discard non-Test Case classes... in future, will inspect class for tests"
        n105 = Unbundle By Name(w287) -> ("Test Project"=w280:path)
        n106 = call "Check if Path Is Test Class.vi"("error in"=w279, "Test Class Path"=w280) -> ("error out"=w282:errorcluster, "TestType"=w281:string, "IsTestObject"=w283:bool)  [unwired: 7 in]
        n107 = case shown="\"TestSuite\"" w281 {
          tunnel: w280 -> [_ w295]
          tunnel: w279 -> [w291 w294]
          tunnel: [w291 w293] -> w278
          tunnel: [_ w292] -> w277
          frame Default {
          }
          frame "TestSuite" {
            # "find all project classes\nwithin TestSuite"
            n108 = call "Get TestSuite Test Paths.vi"("error in (no error)"=w294, "Test Project"=w295) -> ("error out"=w293:errorcluster, "Test Paths"=w292:path[])  [unwired: 8 in]
          }
        }
        n109 = call "Clear All Errors__jki_lib_error_handling -- VI Tester.vi"("error in"=w282) -> ()  [unwired: 4 in, 1 out]
        n110 = Select(t=w280, s=w283, f=path "") -> (s? t:f=w285:path)
        n111 = Build Array (concatenate)(w285, w277) -> (w284:path[])
        n112 = Bundle By Name(cluster=w287, "TestProjectClasses"=w284) -> (w288:T2)
        n113 = call <vilib>:"Add State(s) to Queue__jki_lib_state_machine.vi"("State(s) in (\"\")"=w290) -> ("States Out"=w289:string)  [unwired: 14 in]
      }
      frame "---------- Macro ----------" {
        n114 = call <vilib>:"Add State(s) to Queue__jki_lib_state_machine.vi"("State(s) in (\"\")"=w297) -> ("States Out"=w296:string)  [unwired: 14 in]
      }
      frame "Macro: Load Tree" {
        n115 = call <vilib>:"Add State(s) to Queue__jki_lib_state_machine.vi"("State(s) in Front (\"\")"="Macro: Load Classes\nTest: Load Hierarchy\nSerialize: Store\nTest: Load Tree" ("State(s) in Front"), "State(s) in (\"\")"=w304) -> ("States Out"=w303:string)  [unwired: 13 in]
      }
      frame "Macro: Load Classes" {
        n116 = Unbundle By Name(w308) -> ("Test Project"=w311:path)
        n117 = call <userlib>:"Strip Path Extension - Path__ogtk.vi"("path"=w311) -> ("extension"=w310:string)  [unwired: 1 out]
        n118 = case shown="\"lvclass\"" w310 {
          selector: w310 -> [w318 _ _]
          tunnel: [_ "Project: Get Class\nProject: Get Tests" ("State(s) in Front") "Project: Get Classes\nProject: Get Tests" ("State(s) in Front")] -> w309
          tunnel: w307 -> [w315 w320 w322]
          tunnel: [w314 w320 w322] -> w306
          frame Default {
            w317 = 42 items=["No error", "Argument error", "Memory is full", "Out of zone", "End of file", "File already open", "Generic file I/O error", "File not found", "File permission error", "Disk is full", "Duplicate path", "Too many files open", "System feature not enabled", "Resource file not found", "Cannot add resource", "Resource not found", "Image not found", "Image memory error", "Pen does not exist", "Config type invalid", "Config token not found", "Config parse error", "Config memory error", "Bad external code format", "Bad external code offset", "External code not present", "Null window", "Destroy window error", "Null menu", "Print aborted", "Bad print record", "Print driver error", "Windows error during printing", "Memory error during printing", "Print dialog error", "Generic print error", "Invalid device refnum", "Device not found", "Device parameter error", "Device unit error", "Cannot open device", "Device call aborted", "Generic error", "Cancelled by user", "Object ID too low", "Object ID too high", "Object not in heap", "Unknown heap", "Unknown object (invalid DefProc)", "Unknown object (DefProc not in table)", "Message out of range", "Invalid (null) method", "Unknown message", "Manager call not supported", "Bad address", "Network operation in progress", "Network operation timed out", "Connection is busy", "Network attribute not supported", "Network error", "Address in use", "System out of memory", "Connection aborted", "Connection refused", "Not connected", "Already connected", "Connection closed", "Initialization error (interapplication manager)", "Bad occurrence", "Wait on unbound occurrence handler", "Occurrence queue overflow", "Datalog type conflict", "Unused", "Unrecognized type (interapplication manager)", "Memory corrupt", "Failed to make temporary DLL", "Old CIN version", "Drag socket not found", "Failed to load drop-object", "Failed to register OLE object", "Failed to release OLE object", "Format specifier type mismatch", "Unknown format specifier", "Too few format specifiers", "Too many format specifiers", "Scan failed", "Newer CIN version", "Error converting to variant", "Runtime menu error", "Password tampered", "Variant attribute not found", "Incompatible variant data type", "Event data is not available", "Event Store is not present", "Occurrence is not found", "Event Queue is not created", "Event info is not available", "Refnum passed is NULL", "Error retrieving Class GUID", "Error retrieving CoClass GUID", "Error retrieving TypeLib GUID.", "Bad built application magic bytes.", "Specific driver is different from the specific driver associated with the Logical Name.", "There is no session opened to the class driver.", "Max Error", "MAX - Error with config objects", "MAX - Error loading configuration", "MAX - Group not supported"]
            n119 = Format Into String(format string="Invalid Project Type '%s'", w318) -> (resulting string=w316:string)  [unwired: 2 in, 1 out]
            n120 = call <vilib>:"Error Cluster From Error Code.vi"("error in (no error)"=w315, "error message (\"\")"=w316, "error code (0)"=w317) -> ("error out"=w314:errorcluster)  [unwired: 6 in]
          }
          frame "lvclass" {
          }
          frame "", "lvproj" {
          }
        }
        n121 = call <vilib>:"Add State(s) to Queue__jki_lib_state_machine.vi"("State(s) in (\"\")"=w309) -> ("States Out"=w305:string)  [unwired: 14 in]
        n122 = call <vilib>:"Add State(s) to Queue__jki_lib_state_machine.vi"("State(s) in Front (\"\")"=w305, "State(s) in (\"\")"=w313) -> ("States Out"=w312:string)  [unwired: 13 in]
      }
      frame "Macro: Initialize" {
        n123 = call <vilib>:"Add State(s) to Queue__jki_lib_state_machine.vi"("State(s) in Front (\"\")"="App Data: Initialize" ("State(s) in Front"), "State(s) in (\"\")"=w326) -> ("States Out"=w325:string)  [unwired: 13 in]
      }
      frame "Macro: Run All Tests" {
        # "Run all tests loaded on tree"
        n124 = call <vilib>:"Add State(s) to Queue__jki_lib_state_machine.vi"("State(s) in Front (\"\")"="Serialize: Retrieve\nTest: Run All Tests", "State(s) in (\"\")"=w331) -> ("States Out"=w330:string)  [unwired: 13 in]
      }
      frame "Macro: Run Test Tag" {
        # "used to call \"Graphical Test Runner Support\\Insert Test Loader Cases.vi\" here"
        n125 = call <vilib>:"Add State(s) to Queue__jki_lib_state_machine.vi"("State(s) in Front (\"\")"="Serialize: Retrieve\nTest: Run Test Tag", "State(s) in (\"\")"=w337) -> ("States Out"=w336:string)  [unwired: 13 in]
      }
      frame "Macro: Exit" {
        n126 = call <vilib>:"Add State(s) to Queue__jki_lib_state_machine.vi"("State(s) in Front (\"\")"="App Data: Cleanup\nExit" ("State(s) in Front"), "State(s) in (\"\")"=w341) -> ("States Out"=w340:string)  [unwired: 13 in]
      }
      frame "---------- Serialize ----------" {
        n127 = call <vilib>:"Add State(s) to Queue__jki_lib_state_machine.vi"("State(s) in (\"\")"=w345) -> ("States Out"=w344:string)  [unwired: 14 in]
      }
      frame "Serialize: Store" {
        n128 = Unbundle By Name(w349) -> ("AllTests.TestSuite"=w348:refnum<class "TestSuite.lvclass">)
        n129 = call <userlib>:"Temporary Directory__ogtk.vi"("Relative path (.)"=path "VITester.Cache.obj") -> ("Temporary Directory (+ Relative)"=w353:path)
        n130 = Delete(path (use dialog)=w353) -> (error out=w352:errorcluster)  [unwired: 4 in, 2 out]
        n131 = call <vilib>:"Clear Errors.vi"("error in (no error)"=w352) -> ("error out"=w351:errorcluster)  [unwired: 6 in]
        n132 = Write to Binary File(file (use dialog)=w353, data=w348, error in=w351) -> (error out=w350:errorcluster)  [unwired: 3 in, 2 out]
        n133 = call <vilib>:"Add State(s) to Queue__jki_lib_state_machine.vi"("State(s) in (\"\")"=w356) -> ("States Out"=w355:string)  [unwired: 14 in]
      }
      frame "Serialize: Retrieve" {
        n134 = Unbundle By Name(w358) -> ("AllTests.TestSuite"=w359:refnum<class "TestSuite.lvclass">)
        n135 = call <userlib>:"Temporary Directory__ogtk.vi"("Relative path (.)"=path "VITester.Cache.obj") -> ("Temporary Directory (+ Relative)"=w363:path)
        n136 = Read from Binary File(5:w359, 8:w362, 11:w363) -> (0:w361:errorcluster, 2:w357:refnum<class "TestSuite.lvclass">)  [unwired: 3 in, 2 out]
        n137 = Bundle By Name(cluster=w358, "AllTests.TestSuite"=w357) -> (w360:T2)
        n138 = call <vilib>:"Add State(s) to Queue__jki_lib_state_machine.vi"("State(s) in (\"\")"=w366) -> ("States Out"=w365:string)  [unwired: 14 in]
      }
      frame "---------- For Expansion ----------" {
        n139 = call <vilib>:"Add State(s) to Queue__jki_lib_state_machine.vi"("State(s) in (\"\")"=w368) -> ("States Out"=w367:string)  [unwired: 14 in]
      }
    }
  }
  n140 = Unbundle By Name(w12) -> ("error"=w13:errorcluster)
  n141 = Merge Errors(w13, w14) -> (→"error out":errorcluster)
